vi "Add_Part_of_Track(After_11)_Two_Problems-1.vi"(4 "[IN] Index in subtrack":i32, 5 "[IN] Minimal Sub\ntrack Length":i32, 6 "[IN] Subtrack":T2, 7 "[IN] Indexes for Jumps":i32[](array[numeric]), 8 "error IN":errorcluster, 9 "[IN] Count of variants":i32, 10 "[IN] Subtracks":T1(array[cluster]), 11 "[IN] Still connected\ntracks in group":T3) -> (0 "error OUT":errorcluster, 1 "[OUT] Count of variants":i32, 2 "[OUT] Subtracks":T1(array[cluster]))   [LabVIEW 2013]
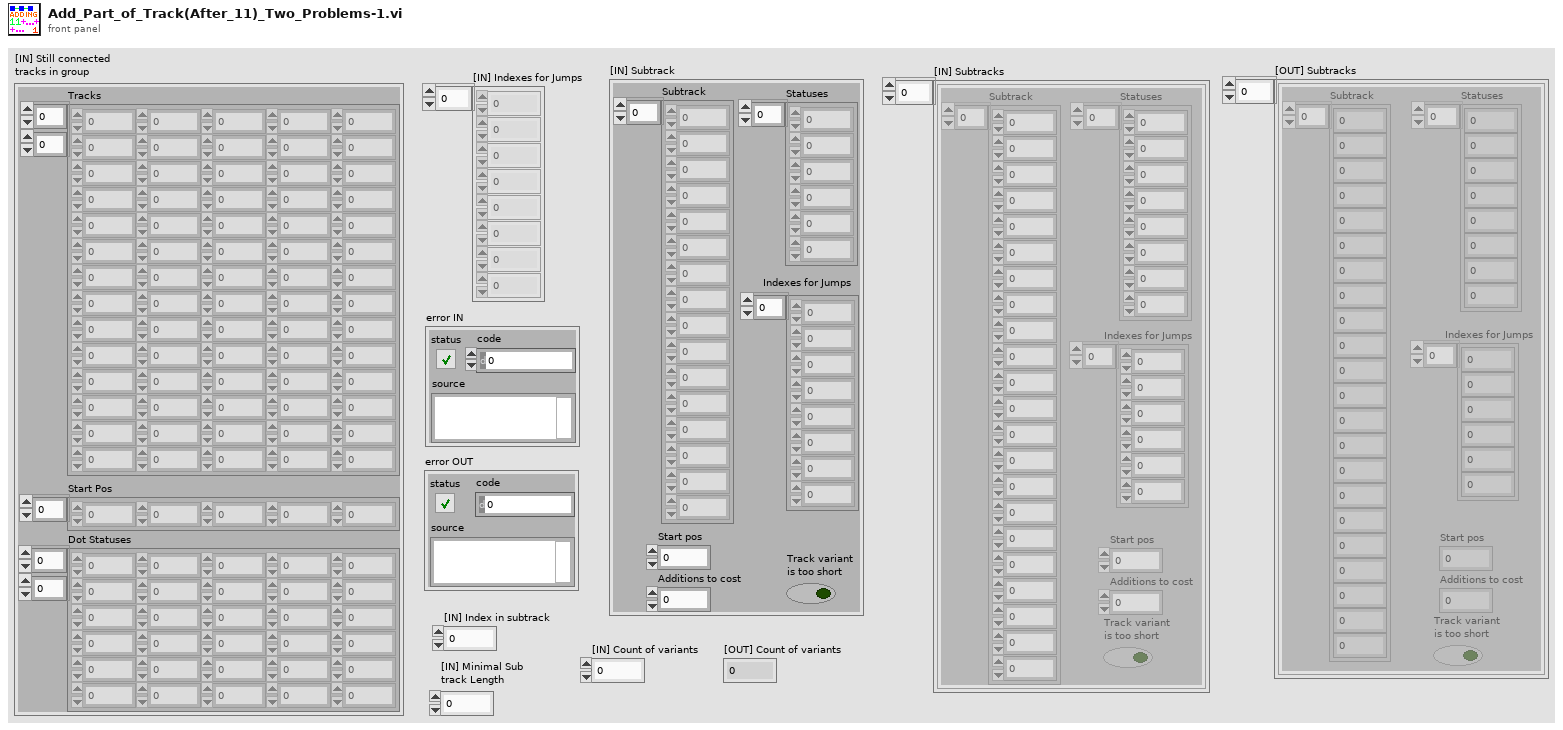
[diagram p1: front panel]
types:
  T1 = cluster{"Subtrack":dbl[], "Statuses":i16[], "Start pos":i32, "Additions to cost":i32, "Track variant \nis too short":bool, "Indexes for Jumps":i32[]}[]
  T2 = cluster{"Subtrack":dbl[], "Statuses":i16[], "Start pos":i32, "Additions to cost":i32, "Track variant \nis too short":bool, "Indexes for Jumps":i32[]}
  T3 = cluster{"Tracks":dbl[][], "Start Pos":i32[], "Dot Statuses":i16[][]}
  T4 = cluster{"Subtrack":dbl[], "Statuses":i16[], "Start pos":i32, "Additions to cost":i8, "Track variant \nis too short":bool, "Indexes for Jumps":i32[]}
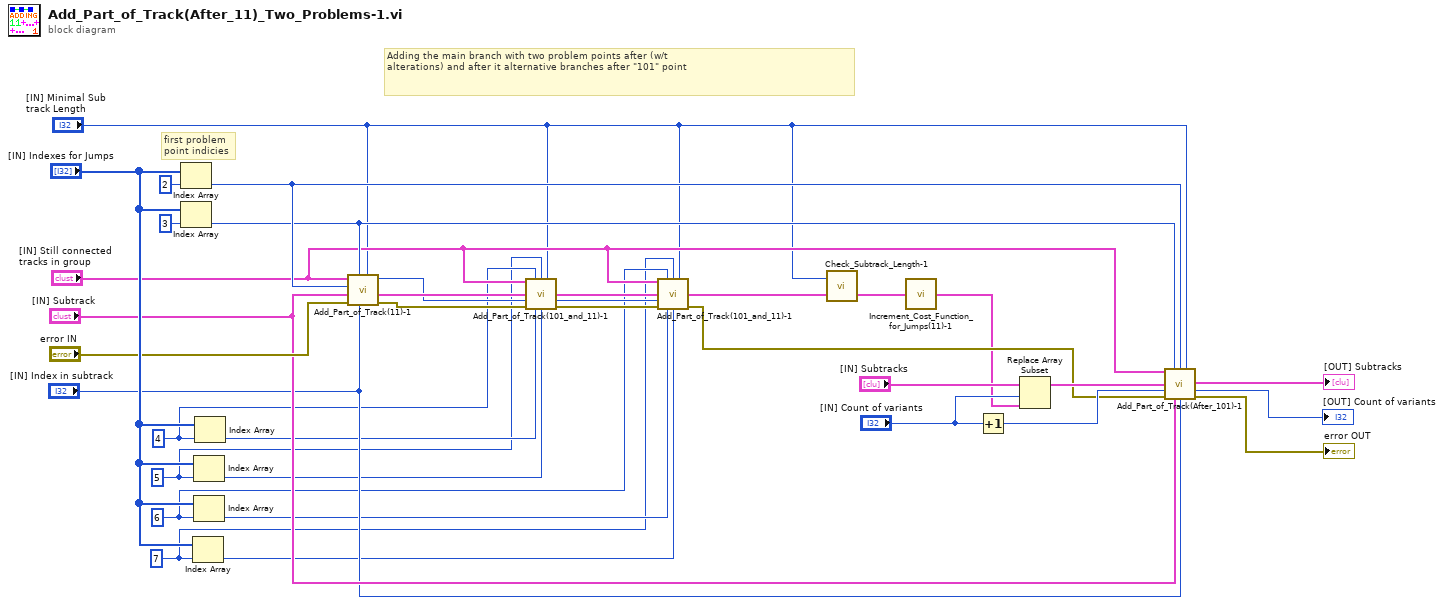
[diagram p0: block diagram]
diagram:
  w3 = 7 ("index")
  w4 = 6 ("index")
  w11 = 5 ("index")
  w12 = 4 ("index")
  # "first problem \npoint indicies"
  # "Adding the main branch with two problem points after (w/t \nalterations) and after it alternative branches after \"101\" point"
  n1 = Index Array(array="[IN] Indexes for Jumps", index=2) -> (element=w22:i32)
  n2 = Index Array(array="[IN] Indexes for Jumps", index=3) -> (element=w21:i32)
  n3 = Index Array(array="[IN] Indexes for Jumps", index=w3) -> (element=w7:i32)
  n4 = Index Array(array="[IN] Indexes for Jumps", index=w11) -> (element=w13:i32)
  n5 = Index Array(array="[IN] Indexes for Jumps", index=w4) -> (element=w10:i32)
  n6 = Index Array(array="[IN] Indexes for Jumps", index=w12) -> (element=w14:i32)
  n7 = call "Add_Part_of_Track(11)-1.vi"("[IN] Minimal Sub\ntrack Length"="[IN] Minimal Sub\ntrack Length", "[IN] Index in subtrack"="[IN] Index in subtrack", "[IN] # of subtrack conta\nining problem point"=w21, "error IN"="error IN", "[IN] Subtrack"="[IN] Subtrack", "[IN] Index of problem\npoint inside subtrack"=w22, "[IN] Still connected\ntracks in group"="[IN] Still connected\ntracks in group") -> ("error OUT"=w15:errorcluster, "[OUT] Subtrack"=w20:T2, "[OUT] Last point in subtrack"=w18:i32)  [unwired: 2 in]
  n8 = call "Add_Part_of_Track(101_and_11)-1.vi"("[IN] Still connected\ntracks in group"="[IN] Still connected\ntracks in group", "[IN] i for Probl\nem  Point Index"=w12, "[IN] i for # of Track \nwith Problem Point"=w11, "[IN] Minimal Sub\ntrack Length"="[IN] Minimal Sub\ntrack Length", "[IN] Subtrack"=w20, "[IN] Index in subtrack"=w18, "error IN"=w15, "[IN] Index of problem\npoint inside subtrack"=w14, "[IN] # of subtrack conta\nining problem point"=w13) -> ("[OUT] Subtrack"=w19:T2, "[OUT] Last point in subtrack"=w17:i32, "error OUT"=w9:errorcluster)  [unwired: 4 in]
  n9 = call "Add_Part_of_Track(101_and_11)-1.vi"("[IN] Still connected\ntracks in group"="[IN] Still connected\ntracks in group", "[IN] i for Probl\nem  Point Index"=w4, "[IN] i for # of Track \nwith Problem Point"=w3, "[IN] Minimal Sub\ntrack Length"="[IN] Minimal Sub\ntrack Length", "[IN] Subtrack"=w19, "[IN] Index in subtrack"=w17, "error IN"=w9, "[IN] Index of problem\npoint inside subtrack"=w10, "[IN] # of subtrack conta\nining problem point"=w7) -> ("[OUT] Subtrack"=w6:T2, "error OUT"=w5:errorcluster)  [unwired: 4 in, 1 out]
  n10 = call "Check_Subtrack_Length-1.vi"("[IN] Subtrack"=w6, "[IN] Minimal Sub\ntrack Length"="[IN] Minimal Sub\ntrack Length") -> ("[OUT] Subtrack"=w2:T4)  [unwired: 1 in]
  n11 = call "Increment_Cost_Function_for_Jumps(11)-1.vi"("[IN] Subtrack"=w2) -> ("[OUT] Subtrack"=w1:T2)
  n12 = Increment(x="[IN] Count of variants") -> (x+1=w30:i32)
  n13 = Replace Array Subset(array="[IN] Subtracks", new element=w1, index="[IN] Count of variants") -> (w31:T1)
  n14 = call "Add_Part_of_Track(After_101)-1.vi"("[IN] Still connected\ntracks in group"="[IN] Still connected\ntracks in group", "[IN] # of subtrack conta\nining problem point"=w21, "[IN] Index of problem\npoint inside subtrack"=w22, "[IN] Minimal Sub\ntrack Length"="[IN] Minimal Sub\ntrack Length", "[IN] Subtracks"=w31, "[IN] Count of variants"=w30, "error IN"=w5, "[IN] Subtrack"="[IN] Subtrack", "[IN] Index in subtrack"="[IN] Index in subtrack") -> ("[OUT] Subtracks"=→"[OUT] Subtracks":T1, "[OUT] Count of variants"=→"[OUT] Count of variants":i32, "error OUT"=→"error OUT":errorcluster)  [unwired: 4 in]
